vi "MPSK.vi"() -> ()   [LabVIEW 2009]
uses:
  <vilib>/Analysis/4window.llb/windowTd.ctl
  <vilib>/addons/Modulation/Analog/MT Downconvert Passband (Real).vi
  <vilib>/measure/maspectr.llb/FFT Power Spectrum for 1 Chan.vi
  <vilib>/addons/Modulation/Analog/MT Upconvert Baseband (Real).vi
  <vilib>/addons/Modulation/Digital/General/MT Generate Bits (Galois, PN Order).vi
  <vilib>/measure/NI_MAPro.lvlib
  <vilib>/Analysis/NI_AALPro.lvlib
panel:
  in  "Tab Control":T1(tab)
  in  "Random Sequence / 1010 Sequence":bool
  in  "Bit Sequence Generation Type\n (Galois PN, Uniform Random)":bool=TRUE
  in  "Visible Bandwidth (Hz)":dbl=6000000000.0 format="%#_6p"
  in  "filter parameter (alpha)":dbl=1.0 format="%.2f"
  in  "pulse shaping filter (none)":T2(ring)=enum."Root Raised Cos"
  in  "frequency offset (Hz)":dbl format="%.2f"
  in  "I DC offset (%)":dbl format="%.2f"
  in  "quadrature skew (deg)":dbl min=-30.0 max=30.0 format="%.2f"
  in  "IQ gain imbalance (dB)":dbl=3.0 format="%.2f"
  in  "Q DC offset (%)":dbl format="%.2f"
  in  "Multitone reference power (dBm)":dbl format="%.2f"
  in  "Multitone tones":cluster{"freq (Hz)":dbl, "amplitude (dB)":dbl}[](array[cluster])=[{"freq (Hz)"=2400000000.0, "amplitude (dB)"=-60.0}] {"amplitude (dB)" format="%.2f"; "freq (Hz)" format="%#.6p"}
  in  "Phase Noise inverse f exponent for noise shape":dbl=1.0 format="%.2p"
  in  "Phase Noise offset frequency (Hz)":dbl=100000.0 format="%.2p"
  in  "Phase noise - noise density (dBc/Hz)":dbl=-87.0 format="%.2p"
  in  "AWGN Eb/N0 (10 dB)":dbl=12.0 format="%.2f"
  in  "Number of Symbol Periods to Show For All Time Domain Graphs":dbl=16.0
  out "Passband Bandwidth":dbl=2400000000.0 format="%#_6p"
  out "Samples per Symbol":i32=60
  out "sampling frequency (Hz)":dbl=72000000000.0 format="%#.6p"
  in  "Number of Symbols (The M in M-PSK) (2, 4, 8, and 16 are valid)":u32=4 min=2 max=16 step=2 format="%.0p"
  in  "symbol rate (Hz)":dbl=1200000000.0 format="%#.6p"
  in  "Phase Noise?":bool
  in  "AWGN?":bool
  in  "IQ Impairments?":bool
  in  "carrier frequency (Hz)":dbl=6000000000.0 min=-0.5 max=0.5 format="%#.6p"
  in  "Multitone Interference?":bool
  in  "Number of Bits to Generate per block":i32=2500 min=256 format="%#.6p"
  out "Recovered Baseband Signal (After matched filtering)":waveform(dbl)[](graph)
  out "Pulse Shaped Baseband Signal":waveform(dbl)[](graph)
  out "Time Domain Passband Signal":waveform(dbl)(graph)
  in  "Passband Time Domain or Passband Frequency Domain?":bool=TRUE
  in  "Center on Passband Spectra?":bool=TRUE
  out "Power spectrum averaged over the number of bits you generate":cluster{"f0":dbl, "df":dbl, "magnitude":dbl[]}(graph)={"f0"=0.0, "df"=471512.77013752464, "magnitude"=[]}
  in  "Constellation \nScale":dbl=1.5 min=1.0
  in  "Show 'ideal' \nTransitions":bool
  in  "Show Actual \nTransitions":bool
  out "Constellation (The grey lines denote 'decision zones' for each symbol)":cluster{dbl[], dbl[]}[](graph)
  out "Bits per Symbol":i32=2
  out "measurements":T3={"frequency offset (Hz)"=14.503155257200888, "frequency drift (Hz)"=-148.4488832792182, "phase offset (deg)"=-0.003712131464084917} {"phase offset (deg)" format="%#.3g"; "frequency drift (Hz)" format="%#.3p"; "frequency offset (Hz)" format="%#.3p"}
  out "Block Number":i32
  out "Symbol Period":dbl=8.333333333333334e-10 format="%#_6p"
  out "Total Bit Errors":i64
  out "Bits simulated so far":i32
  out "BER":dbl
  out "Bit Errors in ths block":i64
  out "Input Bit Stream (first 16)":i8[](array[numeric])
  out "Output Bit Stream (First 16)":i8[](array[numeric])
  in  "Halt Simulation":bool
  in  "Symbol Energy (dBmJ)":dbl format="%#_6p"
  in  "Normal / Offset PSK":bool
  in  "filter length (symbols)":i32=16
  in  "differential PSK":enum16{"disable", "enable"}(ring)
  in  "PN sequence order (Valid range 10-15)":i32=15 min=10 max=15
  # "For a square root raised cosine pulse shape, you end up with a raised cosine pulse shape here. Raised cosine pulse shape,\nyou end up with a square of a raised cosine pulse shape (which isn't a  Nyquist pulse). Triangle waves for no pulse shaping\n(rectangular pulses). Sample at integer multiples of the symbol period and see if that sample is closer to zero or closer to\nsqrt(0.002) to determine if it is a zero or one (maximum likelyhood detection)."
  # "IQ Impairment Parameters"
  # "Channel Impairment Parameters"
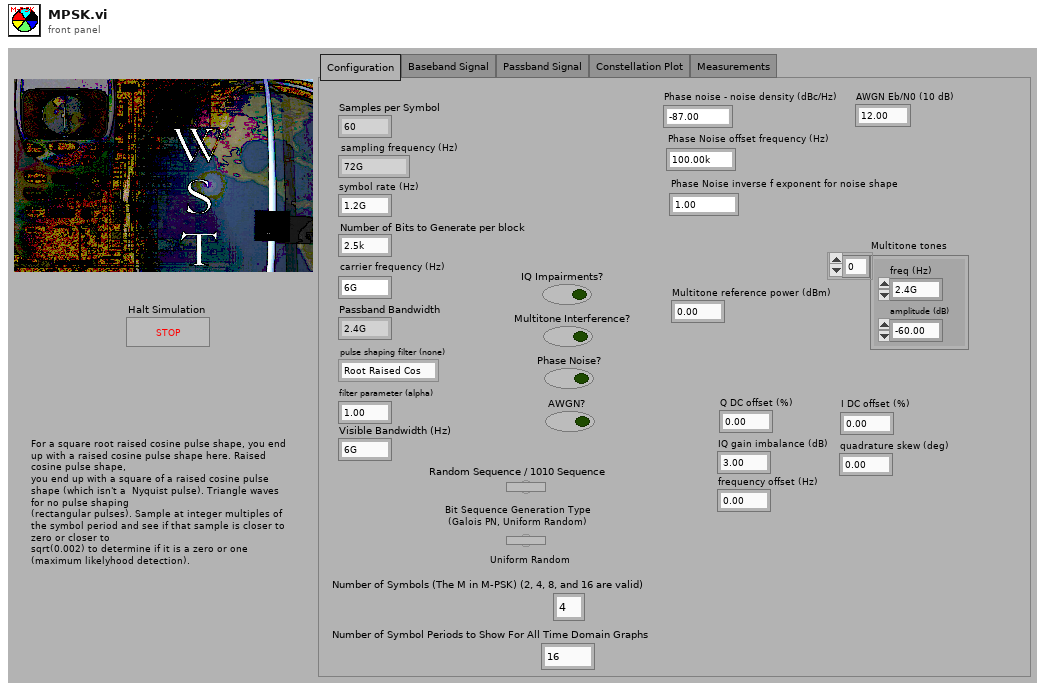
[diagram p1: front panel]
types:
  T1 = enum32{"Configuration", "Baseband Signal", "Passband Signal", "Constellation Plot", "Measurements"}
  T2 = enum16{"none", "Raised Cosine", "Root Raised Cos"}
  T3 = cluster{"frequency offset (Hz)":dbl, "frequency drift (Hz)":dbl, "phase offset (deg)":dbl}
  T4 = cluster{"expected sync location (symbols)":i32, "sync sequence":cdb[], "sync location uncertainty (symbols)":i32, "sync indent (symbols)":i32}
  T5 = cluster{"samples per symbol (16)":i32, "symbol map":cdb[], "differential PSK":enum16{"disable", "enable"}, "PSK type":u16}
  T6 = typedef "NI_AALPro.lvlib/windowTd.ctl" = u32
  T7 = typedef "Complex Data Waveform.ctl" = cluster{"t0":dbl, "dt":dbl, "Y":cdb[]}
  T8 = cluster{"constellation":dbl[], "oversampled data":dbl[]}[]
  T9 = cluster{"constellation":dbl[], "oversampled data":dbl[]}
  T10 = typedef "imagedata.ctl" = cluster{"image type":i32, "image depth":i32, "image":u8[], "mask":u8[], "colors":u32[], "Rectangle":cluster{"left":i16, "top":i16, "right":i16, "bottom":i16}}
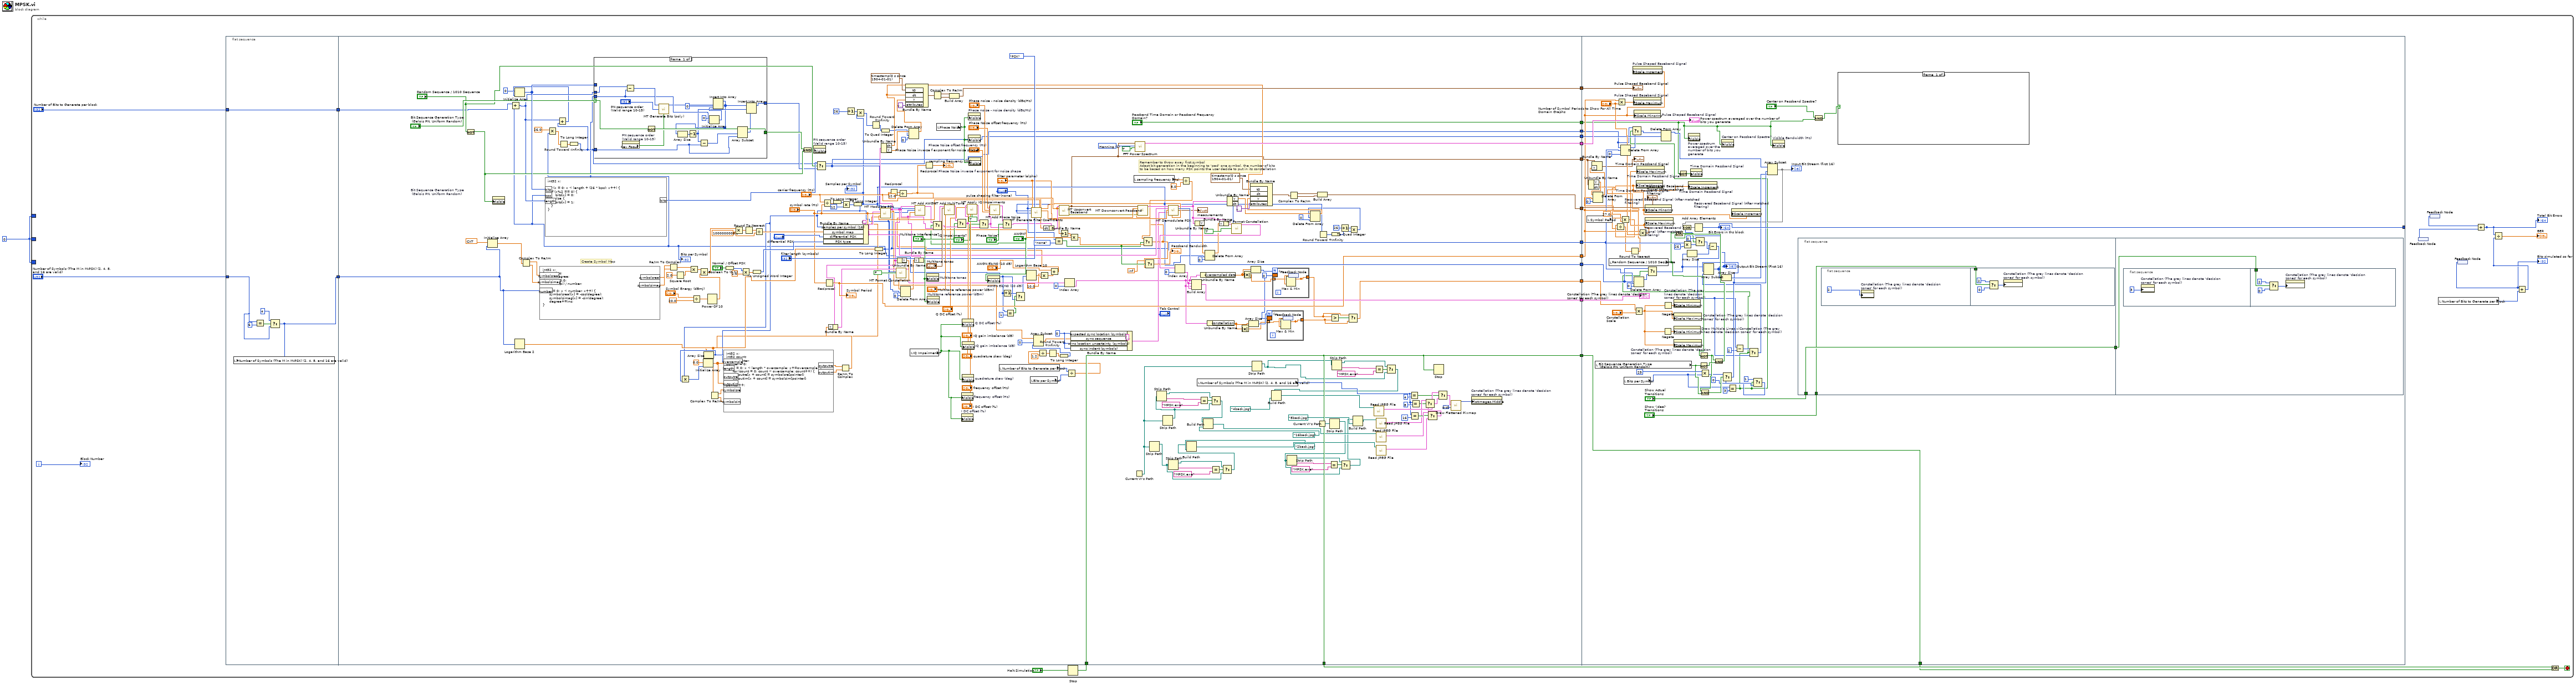
[diagram p0: block diagram]
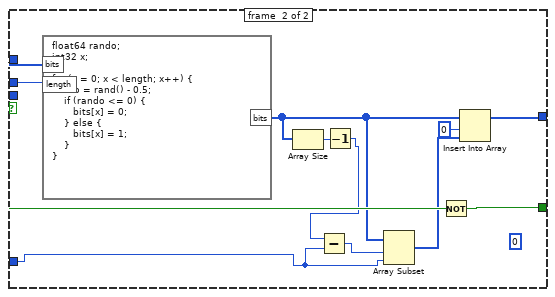
[diagram p2: hidden frame]
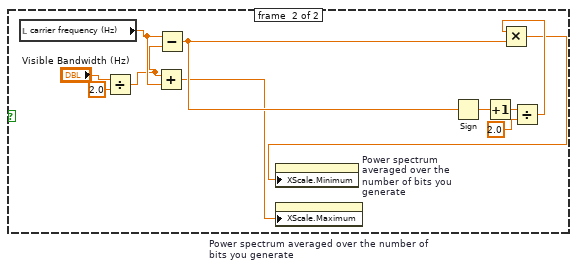
[diagram p3: hidden frame]
diagram:
  w1 = 0
  n1 = while {
    border: w1 -> [_]
    border: w1 -> [_]
    border: w1 -> [_]
    i -> [w19]
    stop <- w8 stop-if-true
    n2 = flat-sequence {
      tunnel: "Number of Symbols (The M in M-PSK) (2, 4, 8, and 16 are valid)" -> [w33]
      tunnel: "Number of Bits to Generate per block" -> [w37]
      tunnel: [w37] -> w5
      tunnel: [w32] -> w4
      tunnel: [w232] -> w31
      tunnel: [w140] -> w30
      tunnel: [w231] -> w29
      tunnel: [w197] -> w28
      tunnel: [w230] -> w27
      tunnel: [w196] -> w26
      tunnel: [w101] -> w23
      tunnel: [w182] -> w22
      tunnel: [w88] -> w20
      tunnel: [w141] -> w10
      tunnel: [w141] -> w11
      tunnel: "Halt Simulation" -> [w141]
      tunnel: [w135] -> w6
      tunnel: w5 -> [w203]
      tunnel: w4 -> [w176]
      tunnel: [w100] -> w3
      tunnel: ["Passband Time Domain or Passband Frequency Domain?"] -> w2
      tunnel: w31 -> [w397]
      tunnel: w30 -> [w329]
      tunnel: w29 -> [w396]
      tunnel: w28 -> [w395]
      tunnel: w27 -> [w331]
      tunnel: w26 -> [w364]
      tunnel: [w384] -> w13
      tunnel: w23 -> [w374]
      tunnel: w22 -> [w391]
      tunnel: w20 -> [w390]
      tunnel: w11 -> [w382]
      tunnel: [w382] -> w9
      tunnel: w6 -> [w381]
      tunnel: w3 -> [w358]
      tunnel: w2 -> [w361]
      frame #0 {
        n3 = Equal?(x=w33, y=u32 6) -> (x = y?=w35:bool)
        n4 = Select(t=u32 4 ("y"), s=w35, f=w33) -> (s? t:f=w32:u32)
        n5 = local write "Number of Symbols (The M in M-PSK) (2, 4, 8, and 16 are valid)"(w32) -> ()
      }
      frame #1 {
        w117 = 0 ("expected sync location (symbols)")
        w92 = 0
        w214 = 1000000000.0 ("y")
        w283 = T6 1 items=["Rectangle"=0, "Hanning"=1, "Hamming"=2, "Blackman-Harris"=3, "Exact Blackman"=4, "Blackman"=5, "Flat Top"=6, "4 Term B-Harris "=7, "7 Term B-Harris"=8, "Low Sidelobe"=9, "Blackman Nuttall"=11, "Triangle"=30, "Kaiser"=60, "Dolph-Chebyshev"=61, "Gaussian"=62] ("window")
        # "Create Symbol Map"
        # "Remember to throw away first symbol\nAdapt bit generation in the beginning to 'pad' one symbol, the number of bits\nto be based on how many PSK points the user decide to put in its constellation"
        n6 = Not(x="Random Sequence / 1010 Sequence") -> (.not. x?=w236:bool)
        n7 = Initialize Array(cxt 0.0+0.0i, w176) -> (w279:cxt[])
        n8 = property on="Bit Sequence Generation Type\n (Galois PN, Uniform Random)" class="Bool (strict)"("Visible"=w236) -> ()  [unwired: 2 in, 2 out]
        n9 = Logarithm Base 2(1:w176) -> (0:w212:dbl)
        n10 = Complex To Re/Im(x + iy=w279) -> (x=w277:ext[], y=w278:ext[])
        n11 = formula code="int32 x;\nfloat64 inc;\nfloat64 degree;\ndegree = 0.0;\ninc = (2 * pi) / number;\n\nfor (x = 0; x < number; x++) {\n      symbolsreal[x] = -cos(degree);\n      symbolsimag[x] = -sin(degree);\n      degree+=inc;\n}"("number"=w176, "symbolsreal"=w277, "symbolsimag"=w278) -> ("symbolsreal"=w280:ext[], "symbolsimag"=w281:ext[])
        n12 = Re/Im To Complex(1:w281, 2:w280) -> (0:w229:cxt[])
        n13 = Square Root(x=2.0) -> (sqrt(x)=w228:dbl)
        n14 = Multiply(x=w229, y=w228) -> (x*y=w223:cxt[])
        n15 = Divide(x="Symbol Energy (dBmJ)", y=20.0) -> (x/y=w224:dbl)
        n16 = Power Of 10(x=w224) -> (10^x=w222:dbl)
        n17 = Multiply(x=w223, y=w222) -> (x*y=w217:cxt[])
        n18 = Boolean To (0,1)(Boolean="Normal / Offset PSK") -> (0, 1=w274:i16)
        n19 = Multiply(x=w217, y=w214) -> (x*y=w216:cxt[])
        n20 = Multiply(x=w274, y=2.0) -> (x*y=w272:dbl)
        n21 = Round To Nearest(number=w216) -> (nearest integer value=w215:cxt[])
        n22 = To Unsigned Word Integer(number=w272) -> (unsigned 16bit integer=w275:u16)
        n23 = Divide(x=w215, y=w214) -> (x/y=w213:cxt[])
        n24 = Divide(x="carrier frequency (Hz)", y="symbol rate (Hz)") -> (x/y=w249:dbl)
        n25 = Reciprocal(x="symbol rate (Hz)") -> (1/x=w196:dbl)
        "Symbol Period" <- w196
        n26 = To Long Integer(number=w249) -> (32bit integer=w250:i32)
        n27 = Multiply(x=w250, y=12) -> (x*y=w157:i32)
        n28 = Increment(x=26) -> (x+1=w127:i32)
        n29 = To Long Integer(number=w157) -> (32bit integer=w132:i32)
        "Samples per Symbol" <- w132
        n30 = Bundle By Name(cluster=T5 {"samples per symbol (16)"=16, "symbol map"=[], "differential PSK"=enum."disable", "PSK type"=0} ("PSK system parameters"), "samples per symbol (16)"=w132, "symbol map"=w213, "differential PSK"="differential PSK", "PSK type"=w275) -> (w146:T5)
        n31 = Multiply(x=w127, y=w132) -> (x*y=w131:i32)
        n32 = Round Toward +Infinity(x=w131) -> (ceil(x): smallest int >= x=w186:i32)
        n33 = To Long Integer(number=w212) -> (32bit integer=w101:i32)
        "Bits per Symbol" <- w101
        n34 = Add(x=w203, y=w101) -> (x+y=w134:i32)
        n35 = Multiply(x=26.0 ("y"), y=w101) -> (x*y=w138:dbl)
        n36 = Round Toward -Infinity(1:w138) -> (0:w139:dbl)
        n37 = To Long Integer(number=w139) -> (32bit integer=w135:i32)
        n38 = Add(x=w134, y=w135) -> (x+y=w133:i32)
        n39 = Initialize Array(i64 0, w133) -> (w269:i64[])
        n40 = formula code="int32 x;\n\nfor (x = 0; x < length + (26 * bps); x++) {\n   if (x%2 == 0) {\n       bits[x] = 0;\n   } else {\n       bits[x] = 1;\n   }\n}"("bits"=w269, "length"=w134, "bps"=w101) -> ("bits"=w237:i64[])
        n41 = case shown="True" "Bit Sequence Generation Type\n (Galois PN, Uniform Random)" {
          selector: "Bit Sequence Generation Type\n (Galois PN, Uniform Random)" -> [w312 w323]
          tunnel: w134 -> [w303 w324]
          tunnel: [w296 w320] -> w136
          tunnel: [w311 w322] -> w234
          tunnel: w269 -> [_ w321]
          tunnel: w101 -> [w306 _]
          tunnel: w135 -> [w301 w319]
          frame #0 {
            n42 = property on="PN sequence order (Valid range 10-15)" class="DigNum (strict)"() -> ("Key Focus"=w309:bool)  [unwired: 2 in, 2 out]
            n43 = Subtract(x=w303, y=w306) -> (x-y=w308:i32)
            n44 = Not(x=w312) -> (.not. x?=w311:bool)
            n45 = call-poly <vilib>:"MT Generate Bits (poly).vi"("total bits (128)"=w308, "PN sequence order (9)"="PN sequence order (Valid range 10-15)", "reset? (T)"=w309) -> ("output bit stream"=w302:i8[])  [unwired: 10 in, 2 out]
            n46 = Initialize Array(0 ("dimension size"), w306) -> (w304:i32[])
            n47 = Insert Into Array(array=w302, index=0, new element=w304) -> (w297:i8[])
            n48 = Array Size(array=w297) -> (size(s)=w299:i32)
            n49 = Decrement(x=w299) -> (x-1=w298:i32)
            n50 = Subtract(x=w298, y=w301) -> (x-y=w295:i32)
            n51 = Array Subset(array=w297, index=w295, length=w301) -> (w300:i8[])
            n52 = Insert Into Array(array=w297, index=w298, new element=w300) -> (w296:i8[])
          }
          frame #1 {
            (unwired) 0
            n53 = formula code="float64 rando;\nint32 x;\n\nfor (x = 0; x < length; x++) {\nrando = rand() - 0.5;\n    if (rando <= 0) {\n       bits[x] = 0;\n    } else {\n       bits[x] = 1;\n    }\n}"("bits"=w321, "length"=w324) -> ("bits"=w318:i64[])
            n54 = Array Size(array=w318) -> (size(s)=w316:i32)
            n55 = Decrement(x=w316) -> (x-1=w315:i32)
            n56 = Subtract(x=w315, y=w319) -> (x-y=w314:i32)
            n57 = Array Subset(array=w318, index=w314, length=w319) -> (w317:i64[])
            n58 = Not(x=w323) -> (.not. x?=w322:bool)
            n59 = Insert Into Array(array=w318, index=0, new element=w317) -> (w320:i64[])
          }
        }
        n60 = And(x=w234, y=w236) -> (x .and. y?=w233:bool)
        n61 = property on="PN sequence order (Valid range 10-15)" class="DigNum (strict)"("Visible"=w233) -> ()  [unwired: 2 in, 2 out]
        n62 = Select(t=w237, s="Random Sequence / 1010 Sequence", f=w136) -> (s? t:f=w140:i64[])
        n63 = To Quad Integer(1:w186) -> (0:w185:i64)
        n64 = Reciprocal(x="carrier frequency (Hz)") -> (1/x=w246:dbl)
        n65 = Divide(x=w246, y=12.0) -> (x/y=w148:dbl)
        n66 = local read "IQ Impairments?"() -> (w266:bool)
        n67 = Reciprocal(x=w148) -> (1/x=→"sampling frequency (Hz)":dbl)
        n68 = property on="Multitone tones" class="Arr (strict)"("Visible"="Multitone Interference?") -> ()  [unwired: 2 in, 2 out]
        n69 = property on="Multitone reference power (dBm)" class="DigNum (strict)"("Visible"="Multitone Interference?") -> ()  [unwired: 2 in, 2 out]
        n70 = local read "Phase Noise?"() -> (w258:bool)
        n71 = property on="frequency offset (Hz)" class="DigNum (strict)"("Visible"=w266) -> ()  [unwired: 2 in, 2 out]
        n72 = property on="I DC offset (%)" class="DigNum (strict)"("Visible"=w266) -> ()  [unwired: 2 in, 2 out]
        n73 = property on="Q DC offset (%)" class="DigNum (strict)"("Visible"=w266) -> ()  [unwired: 2 in, 2 out]
        n74 = property on="quadrature skew (deg)" class="DigNum (strict)"("Visible"=w266) -> ()  [unwired: 2 in, 2 out]
        n75 = property on="IQ gain imbalance (dB)" class="DigNum (strict)"("Visible"=w266) -> ()  [unwired: 2 in, 2 out]
        n76 = property on="Phase noise - noise density (dBc/Hz)" class="DigNum (strict)"("Visible"=w258) -> ()  [unwired: 2 in, 2 out]
        n77 = property on="Phase Noise offset frequency (Hz)" class="DigNum (strict)"("Visible"=w258) -> ()  [unwired: 2 in, 2 out]
        n78 = property on="Phase Noise inverse f exponent for noise shape" class="DigNum (strict)"("Visible"=w258) -> ()  [unwired: 2 in, 2 out]
        n79 = property on="AWGN Eb/N0 (10 dB)" class="DigNum (strict)"("Visible"="AWGN?") -> ()  [unwired: 2 in, 2 out]
        n80 = local read "Number of Bits to Generate per block"() -> (w115:i32)
        n81 = Increment(x=w101) -> (x+1=w105:i32)
        n82 = Equal?(x=w101, y=1 ("index")) -> (x = y?=w102:bool)
        n83 = Select(t=w105, s=w102, f=w101) -> (s? t:f=w106:i32)
        n84 = Logarithm Base 10(1:w106) -> (0:w123:dbl)
        n85 = local read "Bits per Symbol"() -> (w114:i32)
        n86 = call <vilib>:"MT Generate Filter Coefficients.vi"("pulse shaping filter (none)"="pulse shaping filter (none)", "modulation type"=enum16{"FSK", "PSK", "QAM", "MSK", "PAM", "ASK"}."PSK", "pulse shaping samples per symbol (16)"=w132, "matched samples per symbol (16)"=w132, "filter parameter"="filter parameter (alpha)", "filter length (symbols)"="filter length (symbols)") -> ("pulse shaping filter coefficients"=w206:dbl[], "matched filter coefficients"=w207:dbl[])  [unwired: 7 in, 1 out]
        n87 = call <vilib>:"MT Modulate PSK.vi"("input bit stream"=w140, "PSK system parameters"=w146, "symbol rate (Hz)"="symbol rate (Hz)", "pulse shaping filter coefficients"=w206) -> ("output complex waveform"=w160:T7, "symbols out"=w116:cdb[])  [unwired: 9 in, 1 out]
        n88 = Array Size(array=w116) -> (size(s)=w169:i32)
        n89 = Multiply(x=w132, y=w169) -> (x*y=w170:i32)
        n90 = Initialize Array(0.0 ("element"), w170) -> (w166:dbl[])
        n91 = Complex To Re/Im(x + iy=w116) -> (x=w168:dbl[], y=w167:dbl[])
        n92 = formula code="int32 x;\nint32 count;\nint32 pointer;\npointer = 0;\nfor (x = 0; x < length * oversample; x+=oversample) {\n      for (count = 0; count < oversample; count++) {\n      outputre[x + count] = symbolsre[pointer];\n      outputim[x + count] = symbolsim[pointer];\n}\npointer++;\n}"("oversample"=w132, "length"=w169, "outputre"=w166, "symbolsre"=w168, "symbolsim"=w167, "outputim"=w166) -> ("outputre"=w165:dbl[], "outputim"=w164:dbl[])
        n93 = Re/Im To Complex(1:w164, 2:w165) -> (0:w163:cdb[])
        n94 = Bundle By Name(cluster=w160, "Y"=w163) -> (w162:T7)
        n95 = Unbundle By Name(w160) -> ("dt"=w205:dbl, "Y"=w194:cdb[])
        n96 = call <vilib>:"MT Format Constellation.vi"("waveform"=w162, "samples per symbol"=w132, "autoscale"=FALSE) -> ("constellation graph"=w181:T8)  [unwired: 11 in, 1 out]
        n97 = Unbundle By Name(w160) -> ("Y"=w191:cdb[])
        n98 = Delete From Array(array=w191, length=w132, index=0) -> (array with subset deleted=w177:cdb[])  [unwired: 1 out]
        n99 = Delete From Array(array=w194, length=w185, index=0) -> (array with subset deleted=w193:cdb[])  [unwired: 1 out]
        n100 = Bundle By Name("t0"=timestamp(0 s since 1904-01-01), "dt"=w205, "Y"=w193, "attributes"=variant) -> (w286:waveform(cdb))  [unwired: 1 in]
        n101 = Bundle By Name(cluster=w160, "Y"=w177) -> ()  [unwired: 1 out]
        n102 = Complex To Re/Im(x + iy=w286) -> (x=w287:waveform(dbl), y=w288:waveform(dbl))
        n103 = Build Array(w287, w288) -> (w232:waveform(dbl)[])
        n104 = Multiply(x=10.0, y=w123) -> (x*y=w121:dbl)
        n105 = Add(x="AWGN Eb/N0 (10 dB)", y=w121) -> (x+y=w120:dbl)
        n106 = call <vilib>:"MT Add AWGN.vi"("input complex waveform"=w160, "samples per symbol (16)"=w132, "bits per symbol (1)"=w101, "Eb/N0 (10 dB)"=w120) -> ("output complex waveform"=w161:T7)  [unwired: 9 in, 2 out]
        n107 = Select(t=w161, s="AWGN?", f=w160) -> (s? t:f=w241:T7)
        n108 = call <vilib>:"MT Add MultiTone.vi"("input complex waveform"=w241, "tones"="Multitone tones", "reference power (dBm)"="Multitone reference power (dBm)") -> ("output complex waveform"=w238:T7)  [unwired: 11 in, 1 out]
        n109 = Select(t=w238, s="Multitone Interference?", f=w241) -> (s? t:f=w242:T7)
        n110 = call <vilib>:"MT Apply IQ Impairments.vi"("input complex waveform"=w242, "I DC offset (%)"="I DC offset (%)", "Q DC offset (%)"="Q DC offset (%)", "IQ gain imbalance (dB)"="IQ gain imbalance (dB)", "quadrature skew (deg)"="quadrature skew (deg)", "frequency offset (Hz)"="frequency offset (Hz)", "reset? (T)"=TRUE) -> ("output complex waveform"=w239:T7)  [unwired: 7 in, 1 out]
        n111 = Select(t=w239, s="IQ Impairments?", f=w242) -> (s? t:f=w243:T7)
        n112 = call <vilib>:"MT Add Phase Noise.vi"("input complex waveform"=w243, "offset frequency (Hz)"="Phase Noise offset frequency (Hz)", "noise density (dBc/Hz)"="Phase noise - noise density (dBc/Hz)", "inverse f exponent for noise shape"="Phase Noise inverse f exponent for noise shape") -> ("output complex waveform"=w240:T7)  [unwired: 9 in, 2 out]
        n113 = Select(t=w240, s="Phase Noise?", f=w243) -> (s? t:f=w149:T7)
        n114 = Bundle By Name(cluster=w149, "dt"=w148) -> (w248:T7)
        n115 = Equal?(x="pulse shaping filter (none)", y=T2."none") -> (x = y?=w145:bool)
        n116 = call-poly <vilib>:"MT Upconvert Baseband.vi"("baseband waveform (complex)"=w248, "carrier frequency (Hz)"="carrier frequency (Hz)") -> ("passband waveform"=w100:waveform(dbl), "error out"=w218:errorcluster)  [unwired: 12 in]
        n117 = Increment(x="filter parameter (alpha)") -> (x+1=w210:dbl)
        n118 = Index Array(array=w181, index=0) -> (element=w96:T9)
        n119 = Divide(x=w115, y=w114) -> (x/y=w111:dbl)
        n120 = Divide(x=w111, y=1.2) -> (x/y=w110:dbl)
        n121 = Round Toward +Infinity(x=w110) -> (ceil(x): smallest int >= x=w109:dbl)
        n122 = To Long Integer(number=w109) -> (32bit integer=w108:i32)
        n123 = Array Subset(array=w116, index=0, length=w108) -> (w107:cdb[])
        n124 = Multiply(x=w210, y="symbol rate (Hz)") -> (x*y=w153:dbl)
        n125 = Bundle By Name(cluster=T4 {"expected sync location (symbols)"=0, "sync sequence"=[], "sync location uncertainty (symbols)"=0, "sync indent (symbols)"=0} ("synchronization parameters"), "expected sync location (symbols)"=w117, "sync sequence"=w107, "sync location uncertainty (symbols)"=w117, "sync indent (symbols)"=w117) -> (w98:T4)
        n126 = local read "sampling frequency (Hz)"() -> (w152:dbl)
        n127 = Current VI's Path() -> (path=w63:path)
        n128 = call-poly <vilib>:"FFT Power Spectrum.vi"("dB On (F)"=TRUE, "window"=w283, "time signal"=w100) -> ("power spectrum"=w231:cluster{"f0":dbl, "df":dbl, "magnitude":dbl[]})  [unwired: 5 in, 3 out]
        n129 = Strip Path(path=w63) -> (stripped path=w45:path)  [unwired: 1 out]
        n130 = Strip Path(path=w63) -> (stripped path=w53:path)  [unwired: 1 out]
        n131 = Strip Path(path=w53) -> (stripped path=w54:path, name=w57:string)
        n132 = Strip Path(path=w45) -> (stripped path=w59:path, name=w62:string)
        n133 = Divide(x=w152, y=8.0) -> (x/y=w150:dbl)
        n134 = Select(t=w150, s=w145, f=w153) -> (s? t:f=w144:dbl)
        n135 = call-poly <vilib>:"MT Downconvert Passband.vi"("Waveform"=w100, "carrier frequency (Hz)"="carrier frequency (Hz)", "passband bandwidth (Hz)"=w144, "error in (no error)"=w218) -> ("downconverted waveform (complex baseband)"=w178:T7)  [unwired: 8 in, 3 out]
        n136 = Select(t=inf, s=w145, f=w144) -> (s? t:f=→"Passband Bandwidth":dbl)
        n137 = call <vilib>:"MT Demodulate PSK.vi"("input complex waveform"=w178, "PSK system parameters"=w146, "matched filter coefficients"=w207, "synchronization parameters"=w98, "pulse shaping filter coefficients"=w206) -> ("recovered complex waveform"=w172:T7, "output bit stream"=w230:i8[], "measurements"=→"measurements":T3)  [unwired: 6 in, 2 out]
        n138 = Unbundle By Name(w172) -> ("Y"=w188:cdb[])
        n139 = local read "Number of Symbols (The M in M-PSK) (2, 4, 8, and 16 are valid)"() -> (w73:u32)
        n140 = Equal?(x=w57, y="MPSK.exe") -> (x = y?=w55:bool)
        n141 = Unbundle By Name(w96) -> ("oversampled data"=w175:dbl[])
        n142 = Delete From Array(array=w188, length=w132, index=0) -> (array with subset deleted=w187:cdb[])  [unwired: 1 out]
        n143 = Unbundle By Name(w96) -> ("constellation"=w95:dbl[])
        n144 = Select(t=w54, s=w55, f=w53) -> (s? t:f=w52:path)
        n145 = Build Path(base path=w52, name or relative path=path "16back.jpg" ("path to JPEG file")) -> (appended path=w67:path)
        n146 = Equal?(x=w62, y="MPSK.exe") -> (x = y?=w60:bool)
        n147 = Bundle By Name(cluster=w172, "Y"=w187) -> (w190:T7)
        n148 = Select(t=w59, s=w60, f=w45) -> (s? t:f=w58:path)
        n149 = Build Path(base path=w58, name or relative path=path "2back.jpg" ("path to JPEG file")) -> (appended path=w65:path)
        n150 = Unbundle By Name(w172) -> ("Y"=w199:cdb[])  [unwired: 1 out]
        n151 = call <vilib>:"MT Format Constellation.vi"("waveform"=w190, "samples per symbol"=w132, "autoscale"=TRUE) -> ("constellation graph"=w179:T8)  [unwired: 11 in, 1 out]
        n152 = Index Array(array=w179, index=0) -> (element=w119:T9)
        n153 = Build Array(w96, w119, w96, w119) -> (w182:T8)
        n154 = Absolute Value(x=w95) -> (abs(x)=w93:dbl[])
        n155 = Absolute Value(x=w175) -> (abs(x)=w97:dbl[])
        n156 = Array Size(array=w95) -> (size(s)=w94:i32)
        n157 = Array Size(array=w175) -> (size(s)=w174:i32)
        n158 = Strip Path(path=w63) -> (stripped path=w47:path)  [unwired: 1 out]
        n159 = for {
          N: w94 -> [_]
          tunnel: w93 -> [w290] mode=indexing
          tunnel: [w289] -> w90
          border: w92 -> [_]
          n160 = feedback #1() -> (w291:dbl)
          n161 = Max & Min(x=w290, y=w291) -> (max(x,y)=w289:dbl)  [unwired: 1 out]
        }
        n162 = for {
          N: w174 -> [_]
          tunnel: w97 -> [w293] mode=indexing
          tunnel: [w292] -> w89
          border: w92 -> [_]
          n163 = feedback #2() -> (w294:dbl)
          n164 = Max & Min(x=w293, y=w294) -> (max(x,y)=w292:dbl)  [unwired: 1 out]
        }
        n165 = Current VI's Path() -> (path=w70:path)
        n166 = Round Toward +Infinity(x=w132) -> (ceil(x): smallest int >= x=w183:i32)
        n167 = Strip Path(path=w70) -> (stripped path=w38:path)  [unwired: 1 out]
        n168 = Strip Path(path=w38) -> (stripped path=w39:path, name=w44:string)
        n169 = Equal?(x=w44, y="MPSK.exe") -> (x = y?=w42:bool)
        n170 = Greater?(x=w89, y=w90) -> (0:w91:bool)
        n171 = To Quad Integer(1:w183) -> (0:w130:i64)
        n172 = Strip Path(path=w47) -> (stripped path=w48:path, name=w51:string)
        n173 = Increment(x=i64 26) -> (x+1=w125:i64)
        n174 = Select(t=w39, s=w42, f=w38) -> (s? t:f=w41:path)
        n175 = Select(t=w89, s=w91, f=w90) -> (s? t:f=w88:dbl)
        n176 = Multiply(x=w125, y=w130) -> (x*y=w129:i64)
        n177 = Delete From Array(array=w199, length=w129, index=0) -> (array with subset deleted=w198:cdb[])  [unwired: 1 out]
        n178 = Bundle By Name("t0"=timestamp(0 s since 1904-01-01), "dt"=w205, "Y"=w198, "attributes"=variant) -> (w184:waveform(cdb))  [unwired: 1 in]
        n179 = Complex To Re/Im(x + iy=w184) -> (x=w201:waveform(dbl), y=w200:waveform(dbl))
        n180 = Build Array(w201, w200) -> (w197:waveform(dbl)[])
        n181 = Build Path(base path=w41, name or relative path=path "8back.jpg" ("path to JPEG file")) -> (appended path=w40:path)
        n182 = Equal?(x=w51, y="MPSK.exe") -> (x = y?=w49:bool)
        n183 = call <vilib>:"Read JPEG File.vi"("path to JPEG file"=w40) -> ("image data"=w80:T10)  [unwired: 8 in, 2 out]
        n184 = call <vilib>:"Read JPEG File.vi"("path to JPEG file"=w67) -> ("image data"=w84:T10)  [unwired: 8 in, 2 out]
        n185 = call <vilib>:"Read JPEG File.vi"("path to JPEG file"=w65) -> ("image data"=w64:T10)  [unwired: 8 in, 2 out]
        n186 = Select(t=w48, s=w49, f=w47) -> (s? t:f=w46:path)
        n187 = Build Path(base path=w46, name or relative path=path "4back.jpg" ("path to JPEG file")) -> (appended path=w71:path)
        n188 = call <vilib>:"Read JPEG File.vi"("path to JPEG file"=w71) -> ("image data"=w86:T10)  [unwired: 8 in, 2 out]
        n189 = Equal?(x=w73, y=u32 4) -> (x = y?=w75:bool)
        n190 = Equal?(x=w73, y=u32 16) -> (x = y?=w83:bool)
        n191 = Equal?(x=w73, y=u32 8) -> (x = y?=w79:bool)
        n192 = Select(t=w84, s=w83, f=w64) -> (s? t:f=w85:T10)
        n193 = Select(t=w80, s=w79, f=w85) -> (s? t:f=w81:T10)
        n194 = Stop(stop? (T)=w141) -> ()
        n195 = Select(t=w86, s=w75, f=w81) -> (s? t:f=w77:T10)
        n196 = call <vilib>:"Draw Flattened Pixmap.vi"("image data"=w77, "picture"=picture data[5B]) -> ("new picture"=w87:picture)  [unwired: 7 in]
        n197 = property on="Constellation (The grey lines denote 'decision zones' for each symbol)" class="XYGraph (strict)"("PlotImages.Middle"=w87) -> ()  [unwired: 2 in, 2 out]
      }
      frame #2 {
        n198 = local read "Symbol Period"() -> (w356:dbl)
        n199 = Unbundle By Name(w358) -> ("Y"=w360:dbl[], "dt"=w353:dbl)
        n200 = local read "Bit Sequence Generation Type\n (Galois PN, Uniform Random)"() -> (w343:bool)
        n201 = local read "Random Sequence / 1010 Sequence"() -> (w369:bool)
        n202 = Multiply(x=w364, y="Number of Symbol Periods to Show For All Time Domain Graphs") -> (x*y=w394:dbl)
        n203 = Multiply(x=w356, y=27.0) -> (x*y=w354:dbl)
        n204 = Divide(x=w354, y=w353) -> (x/y=w352:dbl)
        n205 = Delete From Array(array=w329, length=w374, index=0) -> (array with subset deleted=w328:i64[])  [unwired: 1 out]
        n206 = local read "Bits per Symbol"() -> (w340:i32)
        n207 = Round To Nearest(number=w352) -> (nearest integer value=w351:dbl)
        n208 = Delete From Array(array=w360, length=w351, index=0) -> (array with subset deleted=w350:dbl[])  [unwired: 1 out]
        n209 = Bundle By Name(cluster=w358, "Y"=w350) -> (→"Time Domain Passband Signal":waveform(dbl))
        n210 = property on="Pulse Shaped Baseband Signal" class="WFGraph (strict)"("XScale.Increment"=w364) -> ()  [unwired: 2 in, 2 out]
        n211 = property on="Pulse Shaped Baseband Signal" class="WFGraph (strict)"("XScale.Maximum"=w394) -> ()  [unwired: 2 in, 2 out]
        n212 = property on="Pulse Shaped Baseband Signal" class="WFGraph (strict)"("XScale.MinorInc"=w364) -> ()  [unwired: 2 in, 2 out]
        n213 = Delete From Array(array=w331, length=w374, index=0) -> (array with subset deleted=w330:i8[])  [unwired: 1 out]
        n214 = Multiply(x=w390, y="Constellation \nScale") -> (x*y=w387:dbl)
        n215 = property on="Time Domain Passband Signal" class="WFGraph (strict)"("XScale.MinorInc"=w364) -> ()  [unwired: 2 in, 2 out]
        n216 = Multiply(x=w364, y="Number of Symbol Periods to Show For All Time Domain Graphs") -> (x*y=w366:dbl)
        n217 = property on="Time Domain Passband Signal" class="WFGraph (strict)"("XScale.Maximum"=w366) -> ()  [unwired: 2 in, 2 out]
        n218 = property on="Recovered Baseband Signal (After matched filtering)" class="WFGraph (strict)"("XScale.MinorInc"=w364) -> ()  [unwired: 2 in, 2 out]
        n219 = property on="Recovered Baseband Signal (After matched filtering)" class="WFGraph (strict)"("XScale.Maximum"=w366) -> ()  [unwired: 2 in, 2 out]
        n220 = Negate(x=w387) -> (-x=w388:dbl)
        n221 = Negate(x=w387) -> (-x=w389:dbl)
        n222 = property on="Constellation (The grey lines denote 'decision zones' for each symbol)" class="XYGraph (strict)"("XScale.Minimum"=w389) -> ()  [unwired: 2 in, 2 out]
        n223 = property on="Constellation (The grey lines denote 'decision zones' for each symbol)" class="XYGraph (strict)"("XScale.Maximum"=w387) -> ()  [unwired: 2 in, 2 out]
        n224 = property on="Draw Multiple Lines.viConstellation (The grey lines denote 'decision zones' for each symbol)" class="XYGraph (strict)"("YScale.Minimum"=w388) -> ()  [unwired: 2 in, 2 out]
        n225 = property on="Constellation (The grey lines denote 'decision zones' for each symbol)" class="XYGraph (strict)"("YScale.Maximum"=w387) -> ()  [unwired: 2 in, 2 out]
        n226 = Not(x=w361) -> (.not. x?=w365:bool)
        n227 = Multiply(x=w374, y=26) -> (x*y=w372:i32)
        n228 = property on="Power spectrum averaged over the number of bits you generate" class="WFGraph (strict)"("Visible"=w361) -> ()  [unwired: 2 in, 2 out]
        n229 = property on="Time Domain Passband Signal" class="WFGraph (strict)"("XScale.Increment"=w364) -> ()  [unwired: 2 in, 2 out]
        n230 = property on="Time Domain Passband Signal" class="WFGraph (strict)"("Visible"=w365) -> ()  [unwired: 2 in, 2 out]
        n231 = Not(x=w343) -> (.not. x?=w349:bool)
        n232 = Not(x=w369) -> (.not. x?=w344:bool)
        n233 = Multiply(x=25, y=w340) -> (x*y=w341:i32)
        n234 = And(x=w344, y=w343) -> (x .and. y?=w342:bool)
        n235 = And(x=w344, y=w349) -> (x .and. y?=w368:bool)
        n236 = Or(x=w369, y=w368) -> (x .or. y?=w367:bool)
        n237 = Select(t=0, s=w367, f=w372) -> (s? t:f=w371:i32)
        n238 = property on="Center on Passband Spectra?" class="Bool (strict)"("Visible"=w361) -> ()  [unwired: 2 in, 2 out]
        n239 = Equal?(x=w340, y=3) -> (x = y?=w326:bool)
        n240 = Select(t=w329, s=w326, f=w328) -> (s? t:f=w327:i64[])
        n241 = Select(t=w331, s=w326, f=w330) -> (s? t:f=w325:i8[])
        n242 = Delete From Array(array=w327, length=w381) -> (array with subset deleted=w380:i64[])  [unwired: 1 in, 1 out]
        n243 = Array Size(array=w325) -> (size(s)=w375:i32)
        n244 = Subtract(x=w375, y=w371) -> (x-y=w333:i32)
        n245 = property on="Recovered Baseband Signal (After matched filtering)" class="WFGraph (strict)"("XScale.Increment"=w364) -> ()  [unwired: 2 in, 2 out]
        n246 = Subtract(x=w333, y=2) -> (x-y=w335:i32)
        n247 = Select(t=w335, s=w326, f=w333) -> (s? t:f=w332:i32)
        n248 = Select(t=1, s=w326, f=0) -> (s? t:f=w336:i32)
        n249 = Select(t=w341, s=w342, f=w336) -> (s? t:f=w347:i32)
        n250 = Array Subset(array=w325, index=w347, length=w332) -> (w345:i8[])
        "Output Bit Stream (First 16)" <- w345
        n251 = Array Size(array=w345) -> (size(s)=w376:i32)
        n252 = Array Subset(array=w380, index=w347, length=w376) -> (w346:i64[])
        "Input Bit Stream (first 16)" <- w346
        n253 = Exclusive Or(1:w345, 2:w346) -> (0:w383:i64[])
        n254 = Add Array Elements(numeric array=w383) -> (sum=w384:i64)
        "Bit Errors in ths block" <- w384
        n255 = property on="Visible Bandwidth (Hz)" class="DigNum (strict)"("Visible"=w361) -> ()  [unwired: 2 in, 2 out]
        n256 = flat-sequence {
          tunnel: "Show 'ideal' \nTransitions" -> [w398]
          tunnel: "Show Actual \nTransitions" -> [w399]
          tunnel: [w399] -> w379
          tunnel: w379 -> [w405]
          frame #0 {
            n257 = flat-sequence {
              tunnel: w398 -> [w402]
              frame #0 {
                n258 = property on="Constellation (The grey lines denote 'decision zones' for each symbol)" class="XYGraph (strict)"("Active Plot"=u32 2) -> ()  [unwired: 2 in, 2 out]
              }
              frame #1 {
                n259 = Select(t=u8 2, s=w402, f=u8 0 ("Plot.Plot Interpolation")) -> (s? t:f=w401:u8)
                n260 = property on="Constellation (The grey lines denote 'decision zones' for each symbol)" class="XYGraph (strict)"("Plot.Plot Interpolation"=w401) -> ()  [unwired: 2 in, 2 out]
              }
            }
          }
          frame #1 {
            n261 = flat-sequence {
              tunnel: w405 -> [w408]
              frame #0 {
                n262 = property on="Constellation (The grey lines denote 'decision zones' for each symbol)" class="XYGraph (strict)"("Active Plot"=u32 3) -> ()  [unwired: 2 in, 2 out]
              }
              frame #1 {
                n263 = Select(t=u8 2, s=w408, f=u8 0 ("Plot.Plot Interpolation")) -> (s? t:f=w407:u8)
                n264 = property on="Constellation (The grey lines denote 'decision zones' for each symbol)" class="XYGraph (strict)"("Plot.Plot Interpolation"=w407) -> ()  [unwired: 2 in, 2 out]
              }
            }
          }
        }
        n265 = And(x="Center on Passband Spectra?", y=w361) -> (x .and. y?=w362:bool)
        n266 = case shown="True" w362 {
          frame #0 {
          }
          frame #1 {
            n267 = local read "carrier frequency (Hz)"() -> (w415:dbl)
            n268 = Divide(x="Visible Bandwidth (Hz)", y=2.0) -> (x/y=w411:dbl)
            n269 = Add(x=w411, y=w415) -> (x+y=w414:dbl)
            n270 = Subtract(x=w415, y=w411) -> (x-y=w421:dbl)
            n271 = property on="Power spectrum averaged over the number of bits you generate" class="WFGraph (strict)"("XScale.Maximum"=w414) -> ()  [unwired: 2 in, 2 out]
            n272 = Sign(1:w421) -> (0:w420:dbl)
            n273 = Increment(x=w420) -> (x+1=w418:dbl)
            n274 = Divide(x=w418, y=2.0) -> (x/y=w417:dbl)
            n275 = Multiply(x=w417, y=w421) -> (x*y=w416:dbl)
            n276 = property on="Power spectrum averaged over the number of bits you generate" class="WFGraph (strict)"("XScale.Minimum"=w416) -> ()  [unwired: 2 in, 2 out]
          }
        }
        "Power spectrum averaged over the number of bits you generate" <- w396
        "Recovered Baseband Signal (After matched filtering)" <- w395
        "Pulse Shaped Baseband Signal" <- w397
        "Constellation (The grey lines denote 'decision zones' for each symbol)" <- w391
      }
    }
    n277 = Stop(stop? (T)="Halt Simulation") -> ()
    n278 = feedback #3() -> (w16:i64)
    n279 = feedback #4() -> (w18:i64)
    n280 = local read "Number of Bits to Generate per block"() -> (w14:i32)
    n281 = feedback #5() -> (w12:i32)
    "Bits simulated so far" <- w12
    n282 = Add(x=w18, y=w16) -> (x+y=w17:i64)
    "Total Bit Errors" <- w17
    n283 = Add(x=w12, y=w14) -> (x+y=w15:i32)
    n284 = Divide(x=w17, y=w15) -> (x/y=→"BER":dbl)
    n285 = Or(x=w10, y=w9) -> (x .or. y?=w8:bool)
    "Block Number" <- w19
  }
